vi "Frequency_Response.vi"() -> ()   [LabVIEW 2015]
uses:
  <instrlib>/Agilent DSO1000 Series/Public/Configure/Configure Trigger (Edge).vi
  <instrlib>/Agilent 34401/Public/Data/Read (Single Point).vi
  <instrlib>/Agilent DSO1000 Series/Agilent DSO1000 Series.lvlib
  <instrlib>/Agilent 34401/Agilent 34401.lvlib
  <instrlib>/Agilent 3352X Series/Agilent 3352X Series.lvlib
panel:
  out "Ao Dmm [V_RMS]":dbl
  out "Ao Scope [V_RMS]":dbl
  out "Ai Scope [V_RMS]":dbl
  out "Ai [V]":dbl=2.0 min=0.0 max=5.0 step=0.01
  out "Filter Time Delay [s]":dbl
  out "Date/time":string
  in  "Names: [CSV]":string
  in  "Delay Time [s]":dbl=1.0 caption="Delay Time (s)"
  out "Mdmm":dbl
  out "Gain (DMM) vs. Frequency":cluster{dbl[], dbl[]}(graph)
  out "Mscope":dbl
  out "Gain  (Scope) vs. Frequency":cluster{dbl[], dbl[]}(graph)
  out "fk [Hz]":dbl
  out "Phase Lag [deg]":dbl
  out "Phase vs. Frequency":cluster{dbl[], dbl[]}(graph)
  in  "Increment [%]":dbl=1.0 min=1.0 max=100.0 step=1.0
  in  "Oscilloscope":refnum<visa-resource-name>
  in  "stop":bool
  in  "DMM":refnum<visa-resource-name>
  in  "Stop Frequency [Hz]":dbl
  in  "Start Frequency [Hz]":dbl=1000.0
  in  "Waveform Function":i32(ring) items=["Sine"=0, "Square"=1, "Ramp"=2, "Noise"=3, "DC"=4, "Triangle"=5, "Pulse"=6, "Sinc"=11, "D-Lorentz"=12, "Gaussian"=13, "Expo Fall"=14, "Expo Rise"=15, "Haversine"=16]
  in  "Amplitude [V]":dbl=2.0 min=0.0 max=5.0 step=0.01
  in  "Waveform Generator":refnum<visa-resource-name>
  # "Set Up:"
  # "User Input:"
  # "Output:"
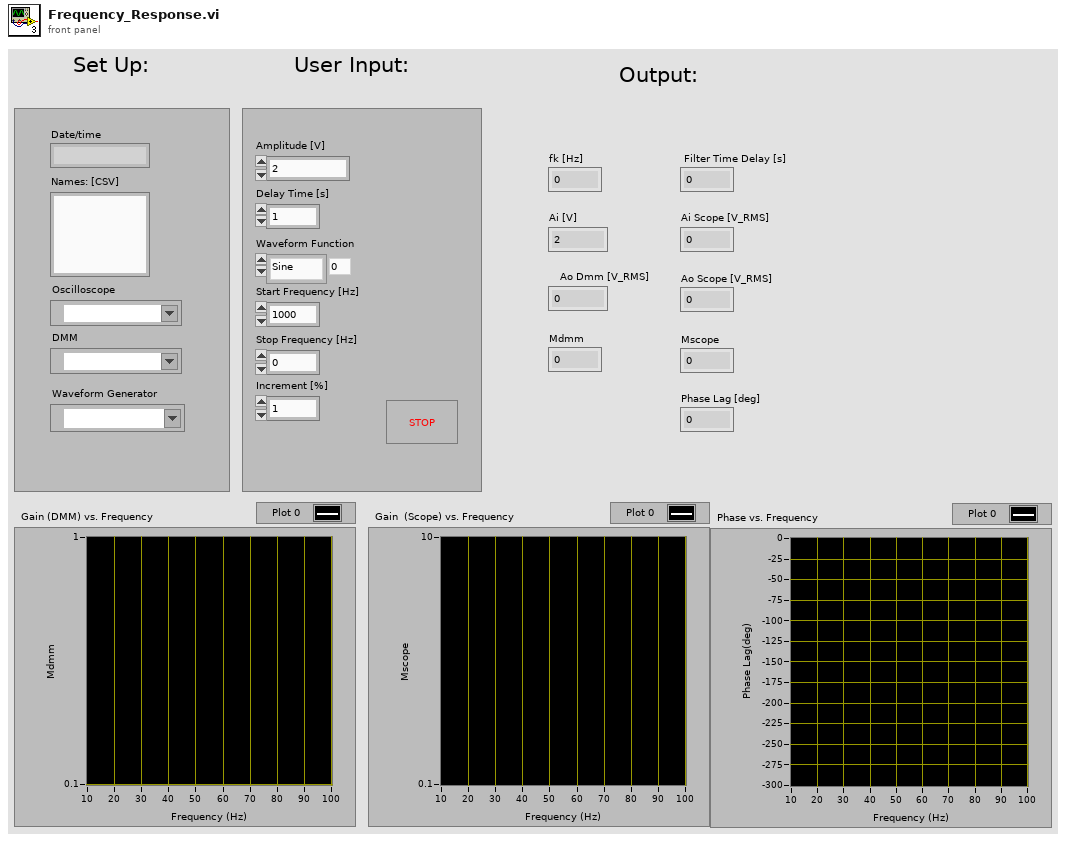
[diagram p1: front panel]
types:
  T1 = enum16{"open", "replace", "create", "open or create", "replace or create", "replace or create with confirmation"}
  T2 = typedef "imagedata.ctl" = cluster{"image type":i32, "image depth":i32, "image":u8[], "mask":u8[], "colors":u32[], "Rectangle":cluster{"left":i16, "top":i16, "right":i16, "bottom":i16}}
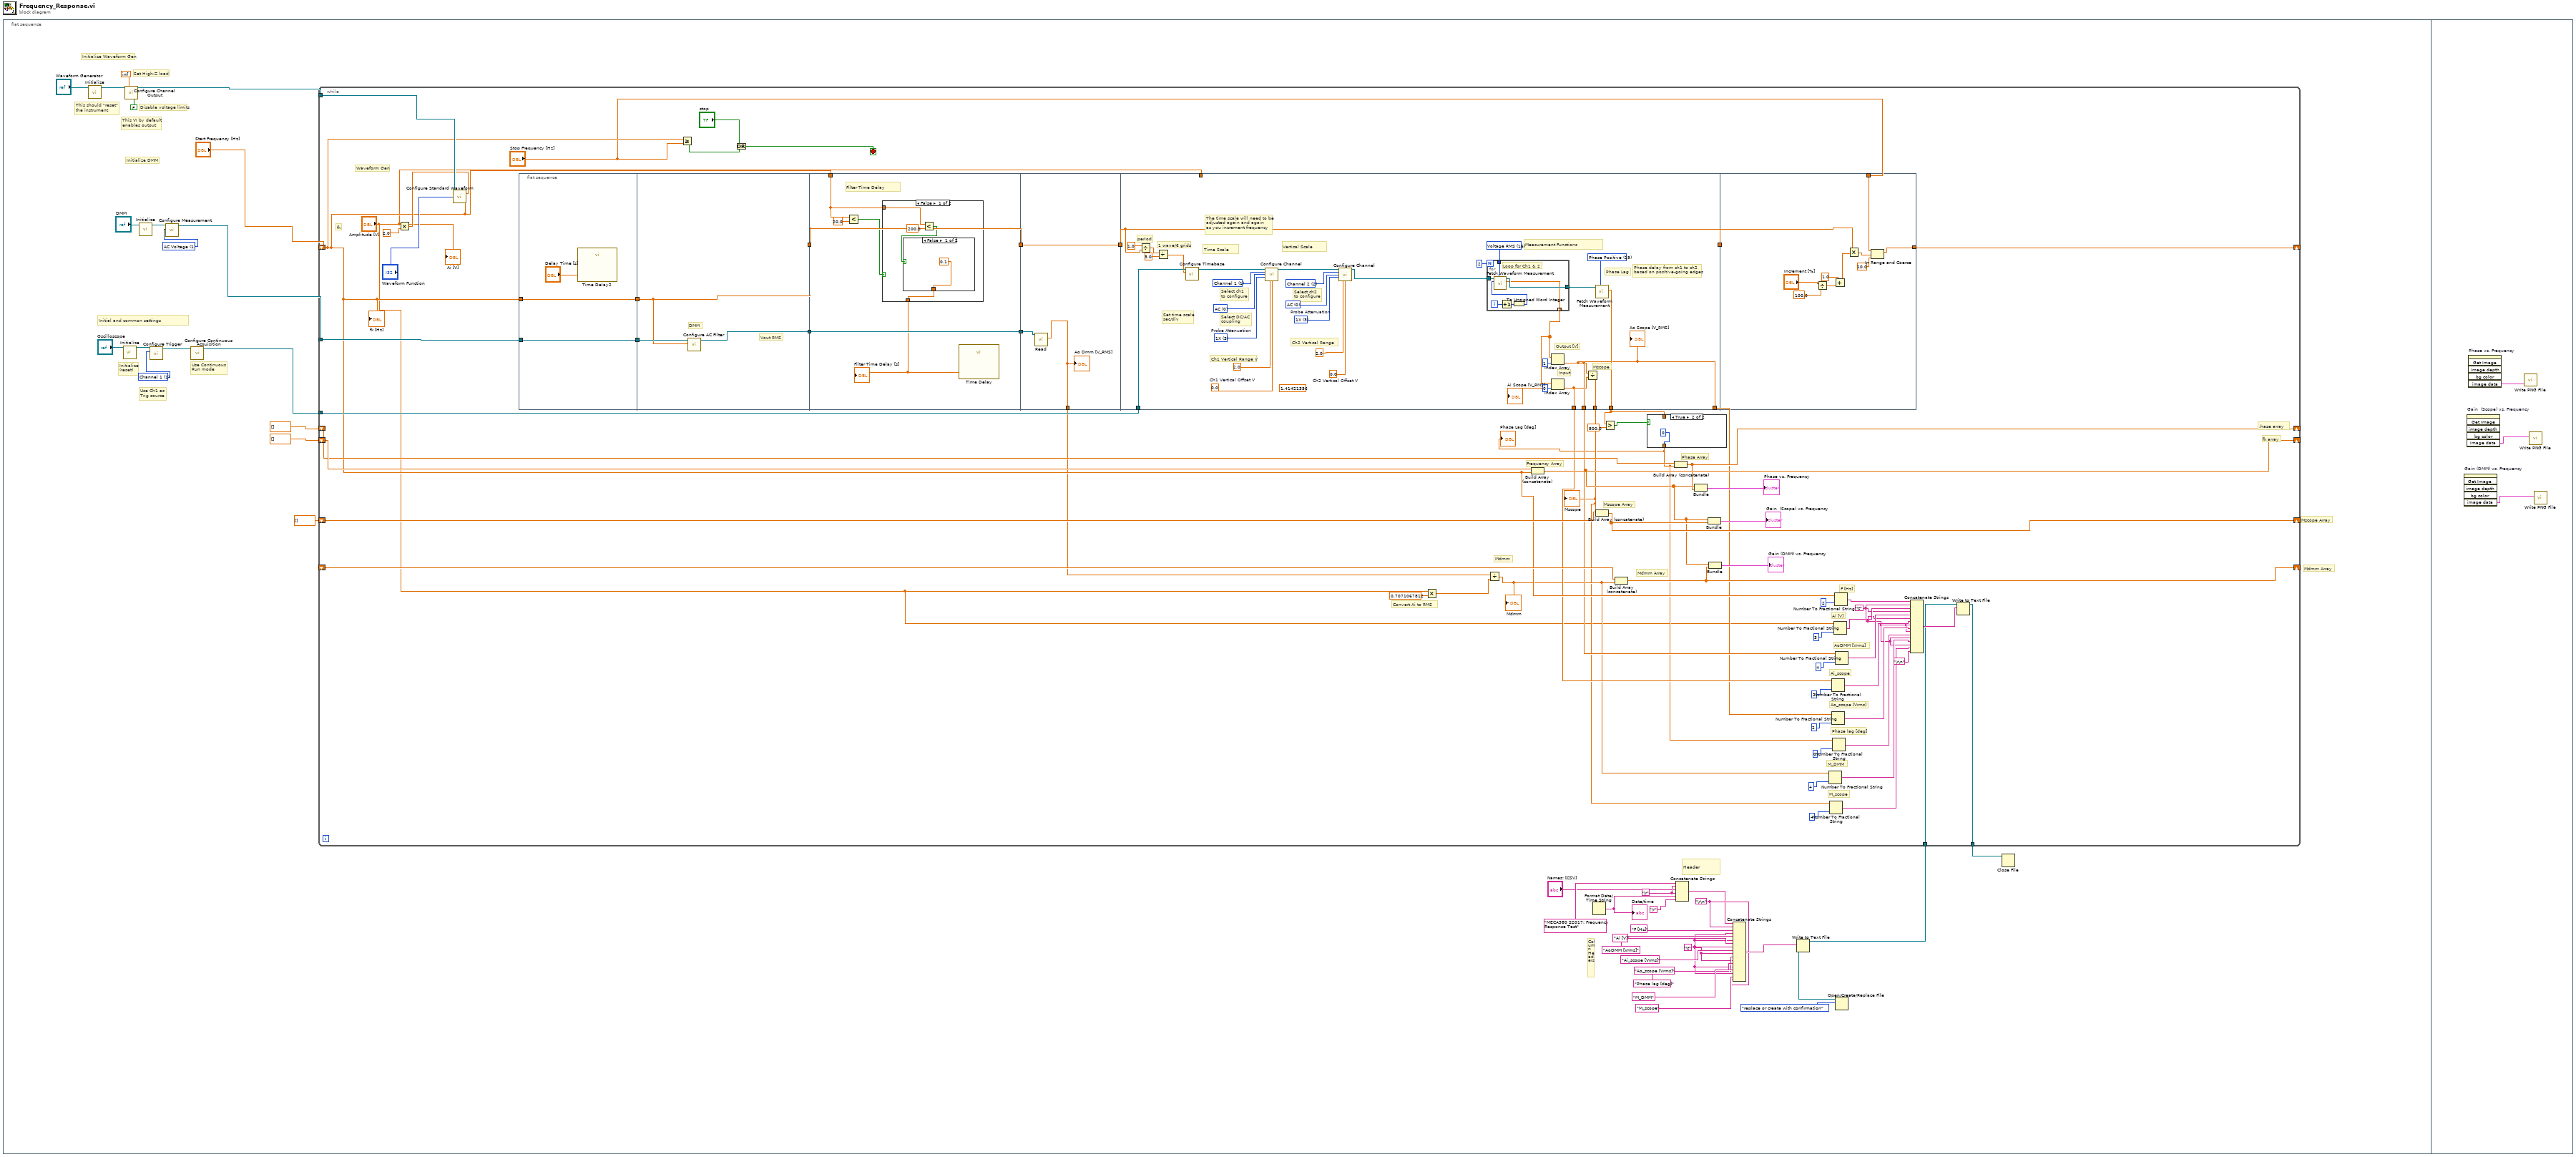
[diagram p0: block diagram]
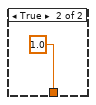
[diagram p3: hidden frame]
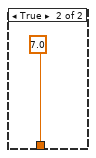
[diagram p4: hidden frame]
diagram:
  n1 = flat-sequence {
    frame #0 {
      w16 = "\r"
      w1 = "\t"
      w2 = "\r\n"
      w27 = u16 1 items=["Channel 1"=1, "Channel 2"=2, "Channel 3"=3, "Channel 4"=4, "External"=5, "External 5"=6, "AC Line"=7] ("Trigger Source (1: Channel 1)")
      w32 = u16 1 items=["DC Voltage", "AC Voltage", "2 - Wire Resistance", "4 - Wire Resistance", "DC Current", "AC Current", "Frequency", "Period", "Continuity", "Diode Checking", "VDC:VDC Ratio", "Temperature", "Capacitance"] ("Function (0: DC Voltage)")
      # "Header"
      # "Column Headers"
      # "Mdmm Array"
      # "Mscope Array"
      # ":hase array"
      # "fk array"
      # "Use Continuous\nRun mode"
      # "Initial and common settings"
      # "Use Ch1 as \nTrig source"
      # "Initialize\n(reset)"
      # "Initialize DMM"
      # "Initialize Waveform Gen"
      # "This VI by default\nenables output"
      # "Disable voltage limits"
      # "Set High-Z load"
      # "This should \"reset\" \nthe instrument"
      n2 = call <instrlib>:"Initialize.vi"("VISA resource name"="Waveform Generator") -> ("VISA resource name out"=w36:refnum<visa-resource-name>)  [unwired: 9 in, 1 out]
      n3 = call <instrlib>:"Initialize.vi"("VISA resource name"="Oscilloscope") -> ("VISA resource name out"=w28:refnum<visa-resource-name>)  [unwired: 9 in, 1 out]
      n4 = call <instrlib>:"Configure Channel Output.vi"("VISA resource name"=w36, "Output Impedance (50 Ohm)"=inf, "Enable Voltage Limit (T: Enable)"=FALSE) -> ("VISA resource name out"=w35:refnum<visa-resource-name>)  [unwired: 11 in, 1 out]
      n5 = call <instrlib>:"Initialize.vi"("VISA resource name"="DMM") -> ("VISA resource name out"=w33:refnum<visa-resource-name>)  [unwired: 9 in, 1 out]
      n6 = call-poly <instrlib>:"Configure Trigger.vi"("VISA resource name"=w28, "Trigger Source (1: Channel 1)"=w27) -> ("VISA resource name out"=w29:refnum<visa-resource-name>)  [unwired: 12 in, 1 out]
      n7 = call <instrlib>:"Configure Measurement.vi"("Function (0: DC Voltage)"=w32, "VISA resource name"=w33) -> ("VISA resource name out"=w31:refnum<visa-resource-name>)  [unwired: 8 in, 1 out]
      n8 = call <instrlib>:"Configure Continuous Acquisition.vi"("VISA resource name"=w29) -> ("VISA resource name out"=w25:refnum<visa-resource-name>)  [unwired: 9 in, 1 out]
      n9 = Format Date/Time String() -> (date/time string=w12:string)  [unwired: 3 in]
      "Date/time" <- w12
      n10 = Concatenate Strings("MECA380 S2017: Frequency Response Test", w16, "Names: [CSV]", w16, w12, "\r") -> (w11:string)
      n11 = Concatenate Strings(w11, w2, "F [Hz]", w1, "Ai [V]", w1, "AoDMM [Vrms]", w1, "Ai_scope [Vrms]", w1, "Ao_scope [Vrms]", w1, "Phase lag [deg]", w1, "M_DMM", w1, "M_scope", w2) -> (w7:string)
      n12 = Open/Create/Replace File(operation (0:open)=T1."replace or create with confirmation" ("Output:")) -> (refnum out=w9:refnum<file>)  [unwired: 5 in, 2 out]
      n13 = Write to Text File(file (use dialog)=w9, text=w7) -> (refnum out=w4:refnum<file>)  [unwired: 2 in, 2 out]
      n14 = while {
        shift-right: [w46] -> _
        shift-left: "Start Frequency [Hz]" -> [w71]
        tunnel: w35 -> [w95]
        tunnel: w31 -> [w104]
        tunnel: w25 -> [w98]
        shift-right: [w83] -> _
        shift-left: dbl[] [] -> [w93]
        shift-right: [w89] -> _
        shift-left: dbl[] [] -> [w92]
        shift-right: [w86] -> _
        shift-left: dbl[] [] -> [w87]
        shift-right: [w82] -> _
        shift-left: _ -> [w84]
        tunnel: w4 -> [w73]
        tunnel: [w50] -> w3
        stop <- w103 stop-if-true
        w48 = "\t"
        # "Convert Ai to RMS"
        # "M_scope"
        # "M_DMM"
        # "Phase lag [deg]"
        # "Ao_scope [Vrms]"
        # "Ai_scope"
        # "AoDMM [Vrms]"
        # "Ai [V]"
        # "F [Hz]"
        # "Frequency Array"
        # "Phase Array"
        # "Mscope Array"
        # "Mdmm Array"
        # "Mdmm"
        # "fk"
        # "Waveform Gen"
        n15 = Multiply(x="Amplitude [V]", y=2.0) -> (x*y=w94:dbl)
        n16 = call <instrlib>:"Configure Standard Waveform.vi"("VISA resource name"=w95, "Amplitude (0.1 Vpp)"=w94, "Waveform Function (0: Sine)"="Waveform Function", "Frequency/Sample Rate/Bandwidth (1000 Hz)"=w71) -> ()  [unwired: 10 in, 2 out]
        n17 = flat-sequence {
          tunnel: w71 -> [w108]
          tunnel: w104 -> [w109]
          tunnel: [w109] -> w80
          tunnel: [w108] -> w79
          tunnel: [w111] -> w100
          tunnel: w80 -> [w112]
          tunnel: w79 -> [w111]
          tunnel: [w110] -> w75
          tunnel: w100 -> [w118]
          tunnel: [w118] -> w78
          tunnel: [w117] -> w76
          tunnel: w75 -> [w117]
          tunnel: w71 -> [w113]
          tunnel: w78 -> [w128]
          tunnel: [w128] -> w77
          tunnel: w76 -> [w127]
          tunnel: [w126] -> w42
          tunnel: w77 -> [w146]
          tunnel: [w146] -> w99
          tunnel: w98 -> [w148]
          tunnel: "Amplitude [V]" -> [_]
          tunnel: [w137] -> w45
          tunnel: [w133] -> w52
          tunnel: [w131] -> w67
          tunnel: [w132] -> w63
          tunnel: [w131] -> w49
          tunnel: w99 -> [w170]
          tunnel: "Stop Frequency [Hz]" -> [w169]
          tunnel: [w166] -> w46
          frame #0 {
            n18 = call "Time Delay2"("Delay Time (s)"="Delay Time [s]") -> ()  [unwired: 10 in, 1 out]
          }
          frame #1 {
            # "Vout RMS"
            # "DMM"
            n19 = call <instrlib>:"Configure AC Filter.vi"("AC Filter Bandwidth (20 Hz)"=w111, "VISA resource name"=w112) -> ("VISA resource name out"=w110:refnum<visa-resource-name>)  [unwired: 8 in, 1 out]
          }
          frame #2 {
            # "Filter Time Delay"
            n20 = Less?(x=w113, y=20.0) -> (x < y?=w115:bool)
            n21 = case shown="False" w115 {
              tunnel: [w119 7.0] -> w114
              tunnel: w113 -> [w121 _]
              frame False {
                n22 = Less?(x=w121, y=200.0) -> (x < y?=w120:bool)
                n23 = case shown="False" w120 {
                  tunnel: [0.1 1.0] -> w119
                  frame False {
                  }
                  frame True {
                  }
                }
              }
              frame True {
              }
            }
            "Filter Time Delay [s]" <- w114
            n24 = call "Time Delay"("Delay Time (s)"=w114) -> ()  [unwired: 10 in, 1 out]
          }
          frame #3 {
            n25 = call-poly <instrlib>:"Read.vi"("VISA resource name"=w127) -> ("Measurement"=w126:dbl)  [unwired: 8 in, 2 out]
            "Ao Dmm [V_RMS]" <- w126
          }
          frame #4 {
            w141 = u16 19 items=["Rise Time", "Fall Time", "Frequency", "Duty Cycle Negative", "Duty Cycle Positive", "Width Negative", "Width Positive", "Over Shoot", "Pre Shoot", "Period", "Amplitude", "Voltage Average", "Voltage Base", "Voltage Max", "Voltage Min", "Voltage Vpp", "Voltage RMS", "Voltage Top", "Phase Negative", "Phase Positive", "Delay Negative", "Delay Positive"] ("Measurement Function (0: Rise Time)")
            w140 = u16 16 items=["Rise Time", "Fall Time", "Frequency", "Duty Cycle Negative", "Duty Cycle Positive", "Width Negative", "Width Positive", "Over Shoot", "Pre Shoot", "Period", "Amplitude", "Voltage Average", "Voltage Base", "Voltage Max", "Voltage Min", "Voltage Vpp", "Voltage RMS", "Voltage Top", "Phase Negative", "Phase Positive", "Delay Negative", "Delay Positive"] ("Measurement Function (0: Rise Time)")
            (unwired) 1.41421356 ("y")
            w154 = 0.0  # Ch2 Vertical Offset V
            w153 = u16 3 items=["0.001X", "0.01X", "0.1X", "1X", "10X", "100X", "1000X"]  # Probe Attenuation
            w152 = u16 0 items=["AC", "DC", "Ground"] ("Vertical Coupling (1: DC)")
            w151 = u16 2 items=["Channel 1"=1, "Channel 2"=2, "Channel 3"=3, "Channel 4"=4] ("Channel (1: Channel 1)")
            w155 = 0.0  # Ch1 Vertical Offset V
            w156 = u16 3 items=["0.001X", "0.01X", "0.1X", "1X", "10X", "100X", "1000X"]  # Probe Attenuation
            w157 = u16 0 items=["AC", "DC", "Ground"] ("Vertical Coupling (1: DC)")
            w158 = u16 1 items=["Channel 1"=1, "Channel 2"=2, "Channel 3"=3, "Channel 4"=4] ("Channel (1: Channel 1)")
            # "Phase Lag"
            # "Ch2 Vertical Range"
            # "Mscope"
            # "Input"
            # "Output [V]"
            # "Measurement Functions"
            # "Phase delay from ch1 to ch2\nbased on positive-going edges"
            # "Ch1 Vertical Range V"
            # "1 wave/6 grids"
            # "period"
            # "Vertical Scale"
            # "Time Scale"
            # "Set time scale\nsec/div"
            # "Select ch2 \nto configure"
            # "Select DC/AC\ncoupling"
            # "Select ch1 \nto configure"
            # "The time scale will need to be \nadjusted again and again\nas you increment frequency"
            n26 = Divide(x=1.0, y=w146) -> (x/y=w145:dbl)
            n27 = Divide(x=w145, y=3.0) -> (x/y=w143:dbl)
            n28 = call <instrlib>:"Configure Timebase.vi"("Timebase (1E-6 s)"=w143, "VISA resource name"=w148) -> ("VISA resource name out"=w149:refnum<visa-resource-name>)  [unwired: 8 in, 1 out]
            n29 = call <instrlib>:"Configure Channel.vi"("VISA resource name"=w149, "Channel (1: Channel 1)"=w158, "Vertical Coupling (1: DC)"=w157, "Probe Attenuation (3: 1X)"=w156, "Vertical Range (10.0 V)"=2.0, "Vertical Offset (0.0 V)"=w155) -> ("VISA resource name out"=w150:refnum<visa-resource-name>)  [unwired: 8 in, 1 out]
            n30 = call <instrlib>:"Configure Channel.vi"("VISA resource name"=w150, "Channel (1: Channel 1)"=w151, "Vertical Coupling (1: DC)"=w152, "Probe Attenuation (3: 1X)"=w153, "Vertical Range (10.0 V)"=2.0, "Vertical Offset (0.0 V)"=w154) -> ("VISA resource name out"=w138:refnum<visa-resource-name>)  [unwired: 8 in, 1 out]
            n31 = for {
              N: 2 -> [_]
              tunnel: w140 -> [w165]
              tunnel: w138 -> [w161]
              tunnel: [w160] -> w139
              tunnel: [w159] -> w135 mode=indexing
              i -> [w164]
              # "Loop for Ch1 & 2"
              n32 = Increment(x=w164) -> (x+1=w163:i32)
              n33 = To Unsigned Word Integer(number=w163) -> (unsigned 16bit integer=w162:u16)
              n34 = call <instrlib>:"Fetch Waveform Measurement.vi"("Measurement Function (0: Rise Time)"=w165, "Source Channel (1: Channel 1)"=w162, "VISA resource name"=w161) -> ("Measurement"=w159:dbl, "VISA resource name out"=w160:refnum<visa-resource-name>)  [unwired: 6 in, 1 out]
            }
            n35 = Index Array(array=w135, index=1) -> (element=w131:dbl)
            "Ao Scope [V_RMS]" <- w131
            n36 = Index Array(array=w135, index=0) -> (element=w132:dbl)
            "Ai Scope [V_RMS]" <- w132
            n37 = Divide(x=w131, y=w132) -> (x/y=w133:dbl)
            n38 = call <instrlib>:"Fetch Waveform Measurement.vi"("Measurement Function (0: Rise Time)"=w141, "VISA resource name"=w139) -> ("Measurement"=w137:dbl)  [unwired: 7 in, 2 out]
          }
          frame #5 {
            n39 = Divide(x="Increment [%]", y=100.0) -> (x/y=w173:dbl)
            n40 = Add(x=1.0, y=w173) -> (x+y=w171:dbl)
            n41 = Multiply(x=w170, y=w171) -> (x*y=w168:dbl)
            n42 = In Range and Coerce(upper limit=w169, x=w168, lower limit=10.0) -> (coerced(x)=w166:dbl)  [unwired: 1 out]
          }
        }
        n43 = Greater Or Equal?(x=w71, y="Stop Frequency [Hz]") -> (x >= y?=w101:bool)
        n44 = Or(x="stop", y=w101) -> (x .or. y?=w103:bool)
        n45 = Multiply(x="Amplitude [V]", y=0.7071067812) -> (x*y=w40:dbl)
        n46 = Divide(x=w42, y=w40) -> (x/y=w56:dbl)
        "Mdmm" <- w56
        n47 = Build Array (concatenate)(w93, w71) -> (w83:dbl[])
        n48 = Build Array (concatenate)(w87, w52) -> (w86:dbl[])
        n49 = Greater?(x=w45, y=800.0) -> (0:w90:bool)
        n50 = Build Array (concatenate)(w84, w56) -> (w82:dbl[])
        n51 = case shown="True" w90 {
          tunnel: [w105 0] -> w44
          tunnel: w45 -> [w105 _]
          frame False {
          }
          frame True {
          }
        }
        "Phase Lag [deg]" <- w44
        n52 = Build Array (concatenate)(w92, w44) -> (w89:dbl[])
        n53 = Bundle(w83, w89) -> (→"Phase vs. Frequency":cluster{dbl[], dbl[]})  [unwired: 1 in]
        n54 = Bundle(w83, w86) -> (→"Gain  (Scope) vs. Frequency":cluster{dbl[], dbl[]})  [unwired: 1 in]
        n55 = Bundle(w83, w82) -> (→"Gain (DMM) vs. Frequency":cluster{dbl[], dbl[]})  [unwired: 1 in]
        n56 = Number To Fractional String(number=w56, precision (6)=i16 4) -> (F-format string=w55:string)  [unwired: 2 in]
        n57 = Number To Fractional String(number=w52, precision (6)=i16 4) -> (F-format string=w53:string)  [unwired: 2 in]
        n58 = Number To Fractional String(number=w49, precision (6)=i16 2) -> (F-format string=w60:string)  [unwired: 2 in]
        n59 = Number To Fractional String(number=w63, precision (6)=i16 2) -> (F-format string=w62:string)  [unwired: 2 in]
        n60 = Number To Fractional String(number=w44, precision (6)=i16 0) -> (F-format string=w58:string)  [unwired: 2 in]
        n61 = Number To Fractional String(number="Amplitude [V]", precision (6)=i16 3) -> (F-format string=w66:string)  [unwired: 2 in]
        n62 = Number To Fractional String(number=w71, precision (6)=i16 2) -> (F-format string=w70:string)  [unwired: 2 in]
        n63 = Number To Fractional String(number=w67, precision (6)=i16 4) -> (F-format string=w65:string)  [unwired: 2 in]
        n64 = Concatenate Strings(w70, w48, w66, w48, w65, w48, w62, w48, w60, w48, w58, w48, w55, w48, w53, "\r\n") -> (w74:string)
        n65 = Write to Text File(file (use dialog)=w73, text=w74) -> (refnum out=w50:refnum<file>)  [unwired: 2 in, 2 out]
        "fk [Hz]" <- w71
        "Mscope" <- w52
        "Ai [V]" <- "Amplitude [V]"
      }
      n66 = Close File(refnum=w3) -> ()  [unwired: 1 in, 2 out]
    }
    frame #1 {
      n67 = invoke on="Gain (DMM) vs. Frequency" class="XYGraph (strict)" method="Get Image"() -> ("image data"=w176:T2)  [unwired: 6 in, 5 out]
      n68 = invoke on="Gain  (Scope) vs. Frequency" class="XYGraph (strict)" method="Get Image"() -> ("image data"=w177:T2)  [unwired: 6 in, 5 out]
      n69 = invoke on="Phase vs. Frequency" class="XYGraph (strict)" method="Get Image"() -> ("image data"=w178:T2)  [unwired: 6 in, 5 out]
      n70 = call <vilib>:"Write PNG File.vi"("image data"=w178) -> ()  [unwired: 9 in, 2 out]
      n71 = call <vilib>:"Write PNG File.vi"("image data"=w177) -> ()  [unwired: 9 in, 2 out]
      n72 = call <vilib>:"Write PNG File.vi"("image data"=w176) -> ()  [unwired: 9 in, 2 out]
    }
  }
